vi "例4.5 显示随机信号波形.vi"() -> ()   [LabVIEW 2017]
panel:
  in  "循环延时":dbl(knob) scale=0.0..10.0
  in  "停止":bool
  out "波形图表":dbl(graph)
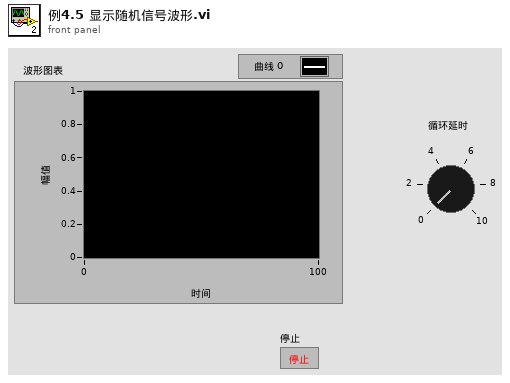
[diagram p1: front panel]
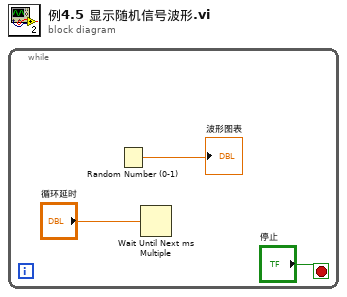
[diagram p0: block diagram]
diagram:
  n1 = while {
    stop <- "停止" stop-if-true
    n2 = Random Number (0-1)() -> (number: 0 to 1=→"波形图表":dbl)
    n3 = Wait Until Next ms Multiple(millisecond multiple="循环延时") -> ()  [unwired: 1 out]
  }
